vi "BRig_RT__Case_Idle__State_Cue_pre__v2.vi"(10 "input_dataExp":u16[](array[numeric]), 11 "input_dataMTrig":u16[](array[numeric])) -> (3 "output_dataMTrig":u16[](array[numeric]), 5 "output_state":T1)   [LabVIEW 2014]
uses:
  myRIO_BRig_RT__Case_NonExp_stateList.ctl
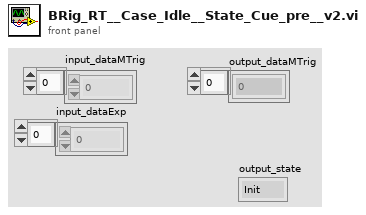
[diagram p1: front panel]
types:
  T1 = typedef "myRIO_BRig_RT__Case_NonExp_stateList.ctl" = enum16{"Init", "UploadSettings_pre", "UploadSettings_Read_dataExp", "UploadSettings_dataExp_1", "UploadSettings_dataExp_2", "UploadSettings_Read_dataLC", "UploadSettings_dataLC_1", "UploadSettings_dataLC_2", "UploadSettings_dataLC_3", "UploadSettings_dataLC_4", "UploadSettings_Read_dataMTrig", "UploadSettings_dataMTrig_1", "UploadSettings_post", "Idle_pre", "IdleEmpty", "IdleEmpty2", "IdleEmpty3", "IdleEmpty4", "Idle", "Idle_2", "Idle_3", "Idle_4", "Idle_5", "Idle_6", "Idle_post", "Cue_pre__pre", "Cue_pre", "Cue", "Cue_LED", "Cue_post", "RewardCalibration_pre", "RewardCalibration", "DispenseWater_pre__pre", "DispenseWater_pre", "DispenseWater", "DispenseWater_post", "TestConnection", "SendData", "Get_FPGA_count_per_ms", "End", "commTCP_connect"}
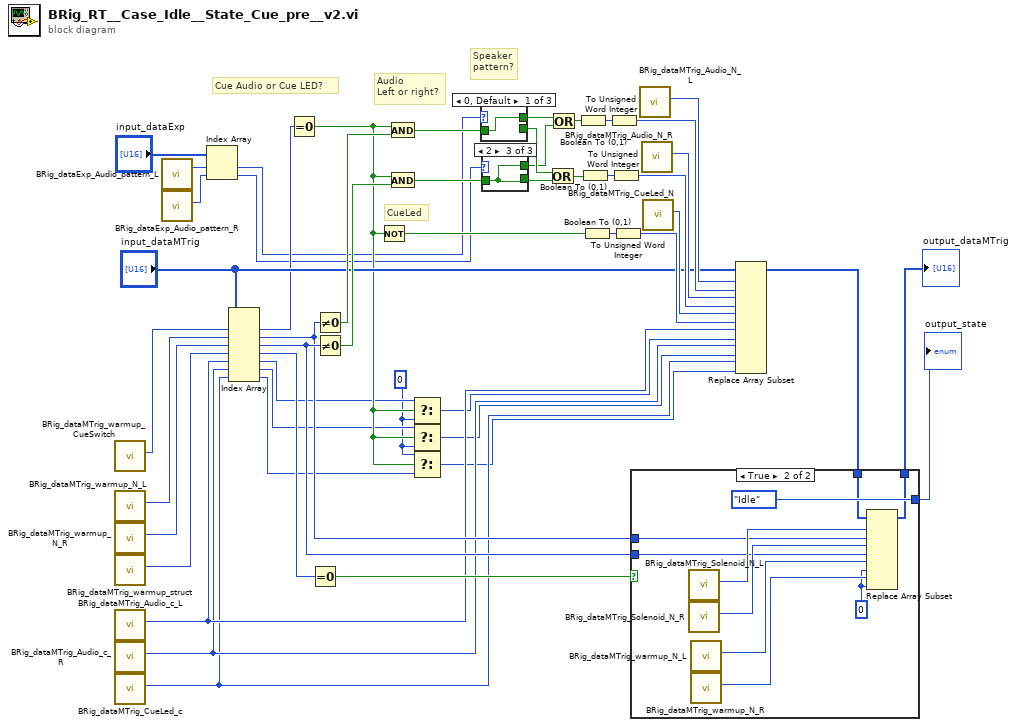
[diagram p0: block diagram]
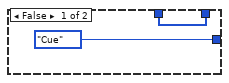
[diagram p2: hidden frame]
diagram:
  w12 = u16 0 ("f")
  # "Speaker\npattern?"
  # "CueLed"
  # "Audio\nLeft or right?"
  # "Cue Audio or Cue LED?"
  n1 = call "BRig_dataMTrig_warmup_CueSwitch.vi"() -> ("output_warmup_CueSwitch"=w18:i32)  [unwired: 11 in]
  n2 = call "BRig_dataMTrig_warmup_N_L.vi"() -> ("output_warmup_N_L"=w49:i32)  [unwired: 11 in]
  n3 = call "BRig_dataMTrig_warmup_N_R.vi"() -> ("output_warmup_N_R"=w48:i32)  [unwired: 11 in]
  n4 = call "BRig_dataMTrig_warmup_struct.vi"() -> ("output_warmup_struct"=w47:i32)  [unwired: 11 in]
  n5 = call "BRig_dataMTrig_Audio_c_L.vi"() -> ("output_Audio_c_L"=w11:i32)  [unwired: 11 in]
  n6 = call "BRig_dataMTrig_Audio_c_R.vi"() -> ("output_Audio_c_R"=w9:i32)  [unwired: 11 in]
  n7 = call "BRig_dataMTrig_CueLed_c.vi"() -> ("output_CueLed_c"=w7:i32)  [unwired: 11 in]
  n8 = call "BRig_dataExp_Audio_pattern_L.vi"() -> ("output_Audio_sp__L"=w3:i32)  [unwired: 11 in]
  n9 = call "BRig_dataExp_Audio_pattern_R.vi"() -> ("output_Audio_sp__R"=w4:i32)  [unwired: 11 in]
  n10 = Index Array(array="input_dataExp", index #1=w3, index #2=w4) -> (element #1=w1:u16, element #2=w2:u16)
  n11 = Index Array(array="input_dataMTrig", index #1=w18, index #2=w49, index #3=w48, index #4=w47, index #5=w11, index #6=w9, index #7=w7) -> (element #1=w17:u16, element #2=w19:u16, element #3=w20:u16, element #4=w28:u16, element #5=w15:u16, element #6=w14:u16, element #7=w13:u16)
  n12 = Equal To 0?(x=w17) -> (x = 0?=w16:bool)
  n13 = Equal To 0?(x=w28) -> (x = 0?=w27:bool)
  n14 = Not Equal To 0?(x=w19) -> (x != 0?=w25:bool)
  n15 = Not Equal To 0?(x=w20) -> (x != 0?=w26:bool)
  n16 = Not(x=w16) -> (.not. x?=w44:bool)
  n17 = And(x=w16, y=w25) -> (x .and. y?=w46:bool)
  n18 = And(x=w16, y=w26) -> (x .and. y?=w45:bool)
  n19 = Select(t=w15, s=w16, f=w12) -> (s? t:f=w10:u16)
  n20 = Select(t=w14, s=w16, f=w12) -> (s? t:f=w8:u16)
  n21 = Select(t=w12, s=w16, f=w13) -> (s? t:f=w6:u16)
  n22 = case shown="0, Default" w1 {
    tunnel: [w50 _ w52] -> w39
    tunnel: [_ w51 w52] -> w40
    tunnel: w46 -> [w50 w51 w52]
    frame 0, Default {
    }
    frame 1 {
    }
    frame 2 {
    }
  }
  n23 = case shown="2" w2 {
    tunnel: [w53 _ w55] -> w38
    tunnel: [_ w54 w55] -> w41
    tunnel: w45 -> [w53 w54 w55]
    frame 0, Default {
    }
    frame 1 {
    }
    frame 2 {
    }
  }
  n24 = Or(x=w40, y=w41) -> (x .or. y?=w37:bool)
  n25 = Or(x=w39, y=w38) -> (x .or. y?=w35:bool)
  n26 = Boolean To (0,1)(Boolean=w35) -> (0, 1=w36:i16)
  n27 = Boolean To (0,1)(Boolean=w37) -> (0, 1=w42:i16)
  n28 = Boolean To (0,1)(Boolean=w44) -> (0, 1=w43:i16)
  n29 = To Unsigned Word Integer(number=w36) -> (unsigned 16bit integer=w31:u16)
  n30 = To Unsigned Word Integer(number=w42) -> (unsigned 16bit integer=w30:u16)
  n31 = To Unsigned Word Integer(number=w43) -> (unsigned 16bit integer=w29:u16)
  n32 = call "BRig_dataMTrig_Audio_N_L.vi"() -> ("output_Audio_N_L"=w34:i32)  [unwired: 11 in]
  n33 = call "BRig_dataMTrig_Audio_N_R.vi"() -> ("output_Audio_N_R"=w33:i32)  [unwired: 11 in]
  n34 = call "BRig_dataMTrig_CueLed_N.vi"() -> ("output_CueLed_N"=w32:i32)  [unwired: 11 in]
  n35 = Replace Array Subset(array="input_dataMTrig", new element #1=w31, index #1=w34, new element #2=w30, index #2=w33, new element #3=w29, index #3=w32, new element #4=w10, index #4=w11, new element #5=w8, index #5=w9, new element #6=w6, index #6=w7) -> (w24:u16[])
  n36 = case shown="True" w27 {
    tunnel: [myRIO_BRig_RT__Case_NonExp_stateList."Cue" ("Enum") myRIO_BRig_RT__Case_NonExp_stateList."Idle" ("Enum")] -> w21
    tunnel: w24 -> [w56 w66]
    tunnel: [w56 w65] -> w22
    tunnel: w20 -> [_ w59]
    tunnel: w19 -> [_ w58]
    frame False {
    }
    frame True {
      w60 = u16 0 ("new element/subarray")
      n37 = call "BRig_dataMTrig_Solenoid_N_L.vi"() -> ("output_Solenoid_N_L"=w64:i32)  [unwired: 11 in]
      n38 = call "BRig_dataMTrig_Solenoid_N_R.vi"() -> ("output_Solenoid_N_R"=w63:i32)  [unwired: 11 in]
      n39 = call "BRig_dataMTrig_warmup_N_L.vi"() -> ("output_warmup_N_L"=w62:i32)  [unwired: 11 in]
      n40 = call "BRig_dataMTrig_warmup_N_R.vi"() -> ("output_warmup_N_R"=w61:i32)  [unwired: 11 in]
      n41 = Replace Array Subset(array=w66, new element #1=w58, index #1=w64, new element #2=w59, index #2=w63, new element #3=w60, index #3=w62, new element #4=w60, index #4=w61) -> (w65:u16[])
    }
  }
  "output_dataMTrig" <- w22
  "output_state" <- w21
